vi "pockelscontrol_MD.vi"() -> ()   [LabVIEW 2012]
uses:
  <vilib>/DAQmx/write.llb/DAQmx Write (Analog DBL 1Chan 1Samp).vi
  GFG/GFGstringGet.vi
  GFG/GFGfpRefGet.vi
  GFG/GFGnumericGet.vi
  <vilib>/DAQmx/create/channels.llb/DAQmx Create Channel (AO-Voltage-Basic).vi
  <vilib>/DAQmx/miscellaneous.llb/DAQmx Fill In Error Info.vi
  GFG/GFG library.lvlib
panel:
  out "error out":errorcluster
  out "Source VI":string
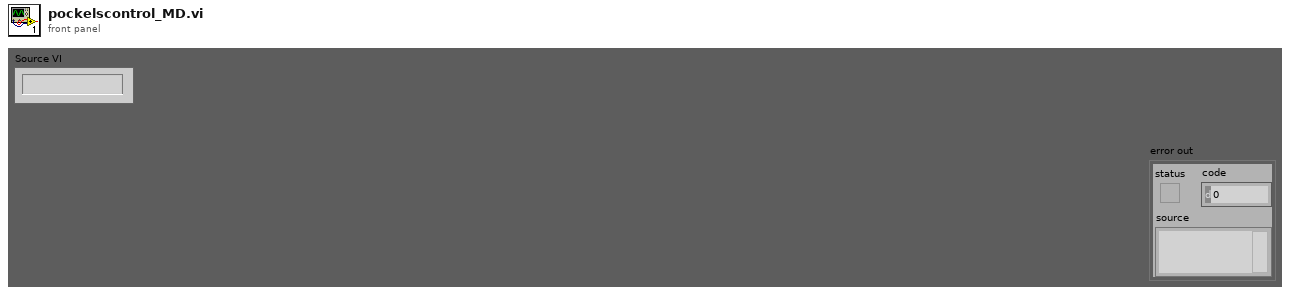
[diagram p1: front panel]
types:
  T1 = enum8{"Enabled", "Disabled", "Disabled and Grayed Out"}
  T2 = cluster{"WaveformChartRef":refnum<vi>, "DigitalRef":refnum<vi>, "ArrayRef":refnum<vi>, "TabControlRef":refnum<vi>, "EnumRef":refnum<vi>, "RingRef":refnum<vi>, "BooleanRef":refnum<vi>, "KnobRef":refnum<vi>, "SlideRef":refnum<vi>, "PathRef":refnum<vi>, "StringRef":refnum<vi>, "ComboBox":refnum<vi>, "WaveformGraphRef":refnum<vi>}
  T3 = enum16{"Left Button", "Center Button", "Right Button", "Window Close"}
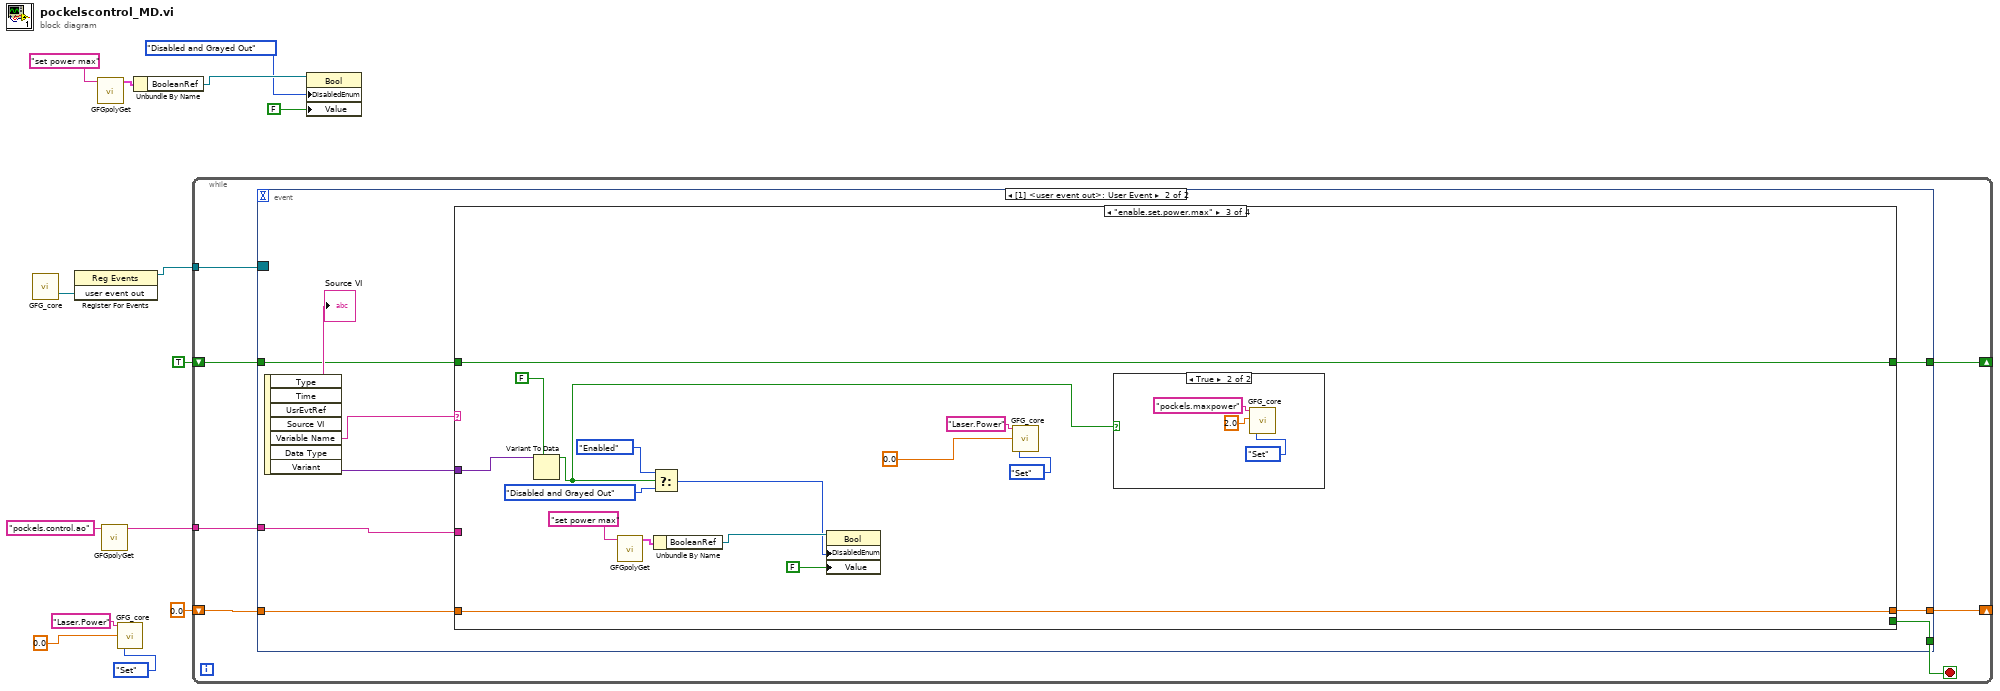
[diagram p0: block diagram]
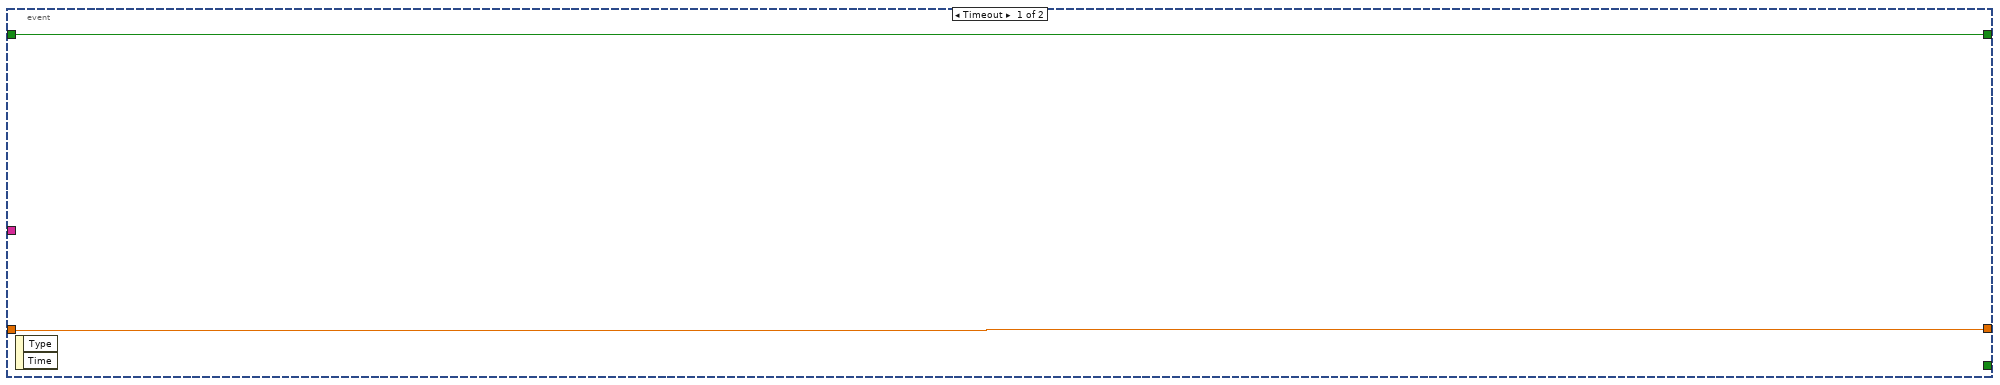
[diagram p2: hidden frame]
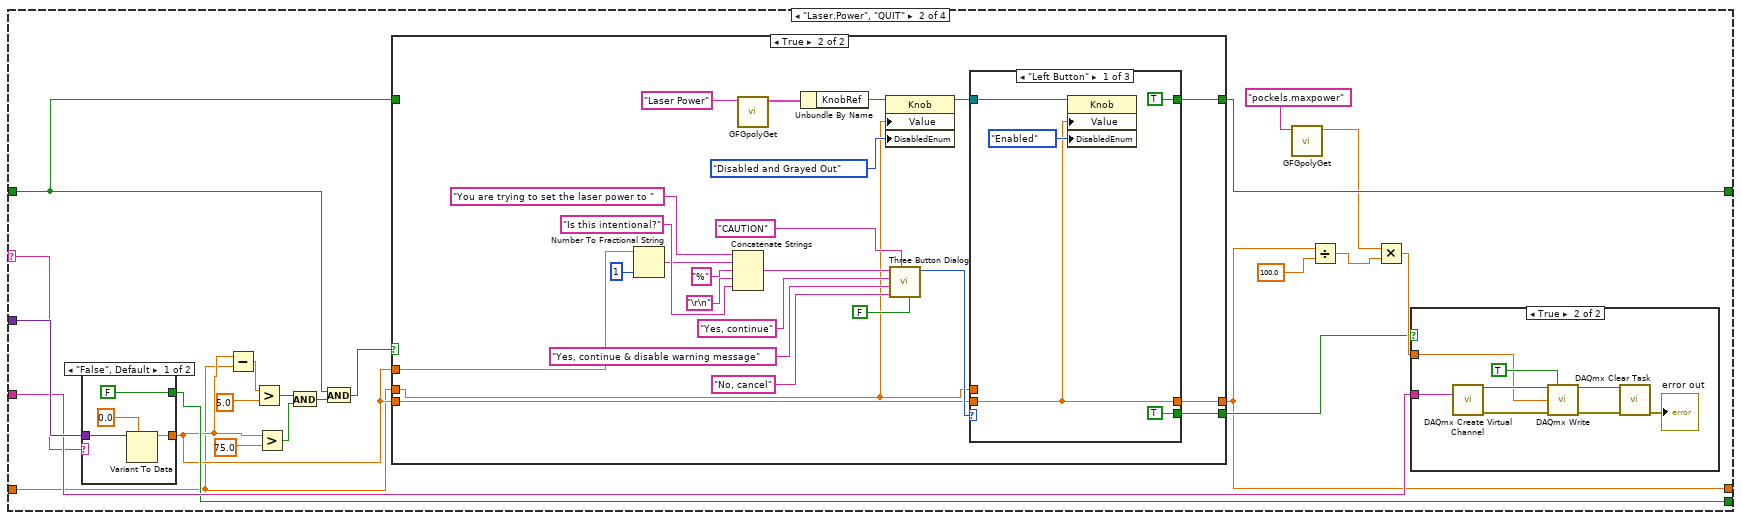
[diagram p4: hidden frame]
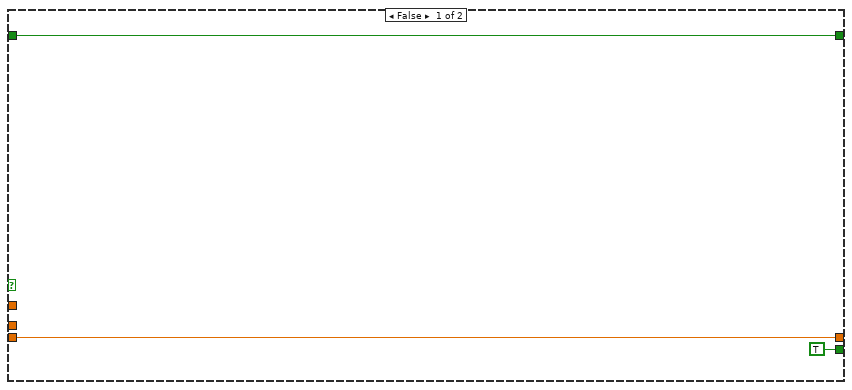
[diagram p5: hidden frame]
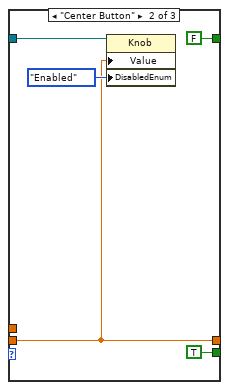
[diagram p6: hidden frame]
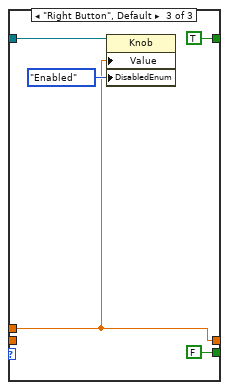
[diagram p7: hidden frame]
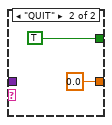
[diagram p9: hidden frame]
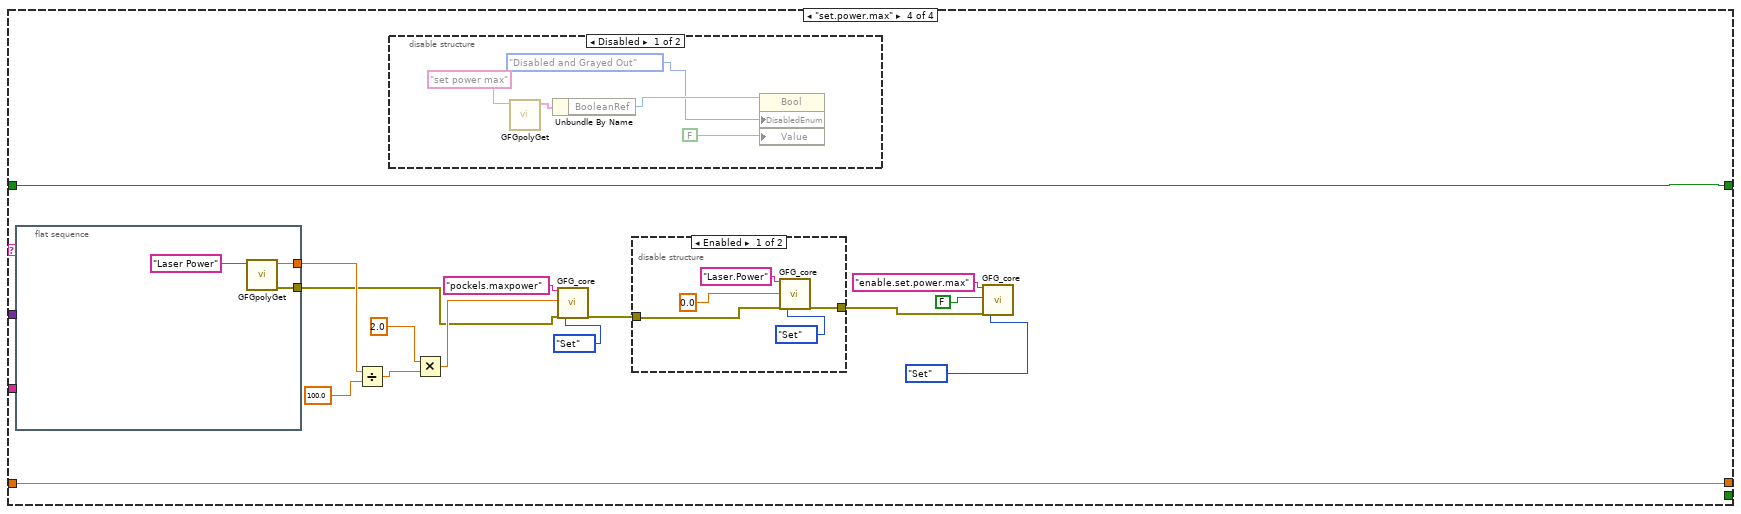
[diagram p11: hidden frame]
diagram:
  n1 = call "GFG_core.vi"() -> ("user event out"=w14:refnum<user-event>)  [unwired: 13 in, 6 out]
  n2 = register-events(w14) -> (reference out=w13:refnum<event-registration>)  [unwired: 2 in, 1 out]
  n3 = call-poly "GFGpolyGet.vi"("Variable Name in"="set power max") -> ("output cluster"=w3:T2)  [unwired: 9 in, 1 out]
  n4 = call-poly "GFGpolyGet.vi"("Variable Name in"="pockels.control.ao" ("Tag in")) -> ("String"=w11:string)  [unwired: 10 in]
  n5 = call "GFG_core.vi"("Variable Name in"="Laser.Power", "Variant in"=0.0 ("Laser Power"), "Action"=enum16{"Init", "Set", "Get"}."Set") -> ()  [unwired: 10 in, 7 out]
  n6 = Unbundle By Name(w3) -> ("BooleanRef"=w4:refnum<vi>)
  n7 = while {
    tunnel: w13 -> [w21]
    tunnel: w11 -> [w19]
    shift-right: [w18] -> _
    shift-left: 0.0 ("Laser Power") -> [w17]
    shift-right: [w16] -> _
    shift-left: TRUE -> [w15]
    stop <- w20 stop-if-true
    n8 = event shown="[1] <user event out>: User Event" {
      selector: w21 -> [_ _]
      dyn-events: _ -> [_ _]
      timeout: _ -> [_ _]
      tunnel: [_ w28] -> w20
      tunnel: w19 -> [_ w30]
      tunnel: [w23 w27] -> w18
      tunnel: w17 -> [w23 w26]
      tunnel: [w22 w25] -> w16
      tunnel: w15 -> [w22 w24]
      event Timeout {
        n9 = event-data() -> ()  [unwired: 1 in, 2 out]
      }
      event User Event {
        n10 = event-data() -> ("Source VI"=→"Source VI":string, "Variable Name"=w32:string, "Variant"=w31:variant)  [unwired: 1 in, 4 out]
        n11 = case shown="\"enable.set.power.max\"" w32 {
          selector: w32 -> [_ w54 _ _]
          tunnel: w31 -> [_ w56 w119 _]
          tunnel: w30 -> [_ w55 _ _]
          tunnel: [_ w53 _ _] -> w28
          tunnel: [w34 w43 w124 w145] -> w27
          tunnel: w26 -> [w34 w40 w124 w145]
          tunnel: [w33 w46 w123 w144] -> w25
          tunnel: w24 -> [w33 w44 w123 w144]
          frame "False", Default {
          }
          frame "Laser.Power", "QUIT" {
            n12 = case shown="\"False\", Default" w54 {
              tunnel: w56 -> [w110 _]
              tunnel: [w109 0.0 ("Laser Power")] -> w41
              tunnel: [FALSE TRUE] -> w53
              frame "False", Default {
                n13 = Variant To Data(type=0.0 ("Laser Power"), Variant=w110) -> (data=w109:dbl)  [unwired: 1 in, 1 out]
              }
              frame "QUIT" {
              }
            }
            n14 = Subtract(x=w41, y=w40) -> (x-y=w39:dbl)
            n15 = Greater?(x=w39, y=5.0) -> (0:w37:bool)
            n16 = Greater?(x=w41, y=75.0) -> (0:w49:bool)
            n17 = And(x=w37, y=w49) -> (x .and. y?=w42:bool)
            n18 = And(x=w44, y=w42) -> (x .and. y?=w45:bool)
            n19 = case shown="True" w45 {
              tunnel: [TRUE w77] -> w47
              tunnel: [w58 w76] -> w46
              tunnel: w44 -> [w58 _]
              tunnel: w40 -> [_ w64]
              tunnel: w41 -> [_ w74]
              tunnel: w41 -> [w57 w65]
              tunnel: [w57 w60] -> w43
              frame False {
              }
              frame True {
                n20 = Number To Fractional String(number=w74, precision (6)=i16 1) -> (F-format string=w63:string)  [unwired: 2 in]
                n21 = Concatenate Strings("You are trying to set the laser power to " ("message"), w63, "%" ("string"), "\r\n", "Is this intentional?" ("string")) -> (w71:string)
                n22 = call-poly "GFGpolyGet.vi"("Variable Name in"="Laser Power") -> ("output cluster"=w69:T2)  [unwired: 9 in, 1 out]
                n23 = Unbundle By Name(w69) -> ("KnobRef"=w68:refnum<vi>)
                n24 = property class="Knob"(reference=w68, "Value"=w64, "DisabledEnum"=T1."Disabled and Grayed Out" ("Disabled")) -> (reference out=w66:refnum<vi>)  [unwired: 1 in, 1 out]
                n25 = call <vilib>:"Three Button Dialog.vi"("Allow user to close window? (TRUE)"=FALSE, "Window Title (\"\")"="CAUTION" ("Window Title (\"\")"), "Right Button Text (\"Cancel\")"="No, cancel" ("Right Button Text (\"Cancel\")"), "Center Button Text (\"No\")"="Yes, continue & disable warning message" ("Center Button Text (\"No\")"), "Left Button Text (\"Yes\")"="Yes, continue" ("Left Button Text (\"Yes\")"), "message"=w71) -> ("Which Button?"=w78:T3)  [unwired: 5 in]
                n26 = case shown="\"Left Button\"" w78 {
                  tunnel: [TRUE TRUE FALSE] -> w77
                  tunnel: [TRUE FALSE TRUE] -> w76
                  tunnel: w66 -> [w85 w90 w95]
                  tunnel: w65 -> [w84 w89 _]
                  tunnel: w64 -> [_ _ w94]
                  tunnel: [w84 w89 w94] -> w60
                  frame "Left Button" {
                    n27 = property class="Knob"(reference=w85, "Value"=w84, "DisabledEnum"=T1."Enabled" ("Disabled")) -> ()  [unwired: 1 in, 2 out]
                  }
                  frame "Center Button" {
                    n28 = property class="Knob"(reference=w90, "Value"=w89, "DisabledEnum"=T1."Enabled" ("Disabled")) -> ()  [unwired: 1 in, 2 out]
                  }
                  frame "Right Button", Default {
                    n29 = property class="Knob"(reference=w95, "Value"=w94, "DisabledEnum"=T1."Enabled" ("Disabled")) -> ()  [unwired: 1 in, 2 out]
                  }
                }
              }
            }
            n30 = call-poly "GFGpolyGet.vi"("Variable Name in"="pockels.maxpower") -> ("Numeric"=w35:dbl)  [unwired: 9 in, 1 out]
            n31 = Divide(x=w43, y=100.0 ("x")) -> (x/y=w52:dbl)
            n32 = Multiply(x=w35, y=w52) -> (x*y=w50:dbl)
            n33 = case shown="True" w47 {
              tunnel: w55 -> [_ w106]
              tunnel: w50 -> [_ w100]
              frame False {
              }
              frame True {
                n34 = call-poly <vilib>:"DAQmx Create Virtual Channel.vi"("physical channels"=w106) -> ("task out"=w105:refnum<k21>, "error out"=w101:errorcluster)  [unwired: 13 in]
                n35 = call-poly <vilib>:"DAQmx Write.vi"("task/channels in"=w105, "auto start"=TRUE, "data"=w100, "error in"=w101) -> ("task out"=w103:refnum<k21>, "error out"=w102:errorcluster)  [unwired: 9 in, 1 out]
                n36 = call <vilib>:"DAQmx Clear Task.vi"("task in"=w103, "error in"=w102) -> ("error out"=→"error out":errorcluster)  [unwired: 13 in]
              }
            }
          }
          frame "enable.set.power.max" {
            n37 = Variant To Data(type=FALSE, Variant=w119) -> (data=w114:bool)  [unwired: 1 in, 1 out]
            n38 = call-poly "GFGpolyGet.vi"("Variable Name in"="set power max") -> ("output cluster"=w126:T2)  [unwired: 9 in, 1 out]
            n39 = Select(t=T1."Enabled" ("Disabled"), s=w114, f=T1."Disabled and Grayed Out" ("Disabled")) -> (s? t:f=w115:T1)
            n40 = Unbundle By Name(w126) -> ("BooleanRef"=w125:refnum<vi>)
            n41 = property class="Bool"(reference=w125, "DisabledEnum"=w115, "Value"=FALSE) -> ()  [unwired: 1 in, 2 out]
            n42 = call "GFG_core.vi"("Variable Name in"="Laser.Power", "Variant in"=0.0 ("Laser Power"), "Action"=enum16{"Init", "Set", "Get"}."Set") -> ()  [unwired: 10 in, 7 out]
            n43 = case shown="True" w114 {
              frame False {
              }
              frame True {
                n44 = call "GFG_core.vi"("Variable Name in"="pockels.maxpower", "Variant in"=2.0 ("Laser Power"), "Action"=enum16{"Init", "Set", "Get"}."Set") -> ()  [unwired: 10 in, 7 out]
              }
            }
          }
          frame "set.power.max" {
            n45 = flat-sequence {
              tunnel: [w152] -> w140
              tunnel: [w151] -> w136
              frame #0 {
                n46 = call-poly "GFGpolyGet.vi"("Variable Name in"="Laser Power") -> ("error out"=w151:errorcluster, "Numeric"=w152:dbl)  [unwired: 9 in]
              }
            }
            n47 = Divide(x=w140, y=100.0 ("x")) -> (x/y=w139:dbl)
            n48 = disable-structure shown="Disabled" {
              frame Disabled {
                n49 = call-poly "GFGpolyGet.vi"("Variable Name in"="set power max") -> ("output cluster"=w157:T2)  [unwired: 9 in, 1 out]
                n50 = Unbundle By Name(w157) -> ("BooleanRef"=w156:refnum<vi>)
                n51 = property class="Bool"(reference=w156, "DisabledEnum"=T1."Disabled and Grayed Out" ("Disabled"), "Value"=FALSE) -> ()  [unwired: 1 in, 2 out]
              }
              frame Enabled {
              }
            }
            n52 = Multiply(x=2.0 ("Laser Power"), y=w139) -> (x*y=w137:dbl)
            n53 = call "GFG_core.vi"("Variable Name in"="pockels.maxpower", "Variant in"=w137, "error in (no error)"=w136, "Action"=enum16{"Init", "Set", "Get"}."Set") -> ("error out"=w135:errorcluster)  [unwired: 9 in, 6 out]
            n54 = disable-structure shown="Enabled" {
              disable-tunnel: w135 -> [w147 _]
              disable-tunnel: [w146 _] -> w132
              frame Enabled {
                n55 = call "GFG_core.vi"("Variable Name in"="Laser.Power", "Variant in"=0.0 ("Laser Power"), "error in (no error)"=w147, "Action"=enum16{"Init", "Set", "Get"}."Set") -> ("error out"=w146:errorcluster)  [unwired: 9 in, 6 out]
              }
              frame Disabled {
              }
            }
            n56 = call "GFG_core.vi"("Variable Name in"="enable.set.power.max", "Variant in"=FALSE, "error in (no error)"=w132, "Action"=enum16{"Init", "Set", "Get"}."Set") -> ()  [unwired: 9 in, 7 out]
          }
        }
      }
    }
  }
  n57 = property class="Bool"(reference=w4, "DisabledEnum"=T1."Disabled and Grayed Out" ("Disabled"), "Value"=FALSE) -> ()  [unwired: 1 in, 2 out]
